vi "PC_DAYWISE.vi"(0 "Refnum in":T1, 1 "BREAKDOWN_STK_HOLD_ID":i32=1, 2 "condition":string="Where BREAKDOWN_DATE between '%s'and '%s' and BREAKDOWN_STK_HOLD_ID ='%d'  ", 5 "Form Date":timestamp, 7 "Array":string[](array[string]), 9 "To Date":timestamp, 11 "error in (no error)":errorcluster, 12 "STATION_ID_CID_TRIGGER":i32) -> (4 "Refnum out":T1, 6 "Count out":string[](array[string]), 15 "error out":errorcluster)   [LabVIEW 2017]
uses:
  <vilib>/addons/database/Connection.llb/Conn ObjectReference.ctl
  <vilib>/addons/database/NI_Database_API.lvlib
panel:
  out "subarray":string[](array[string])
  out "Table":string[][](array[string])
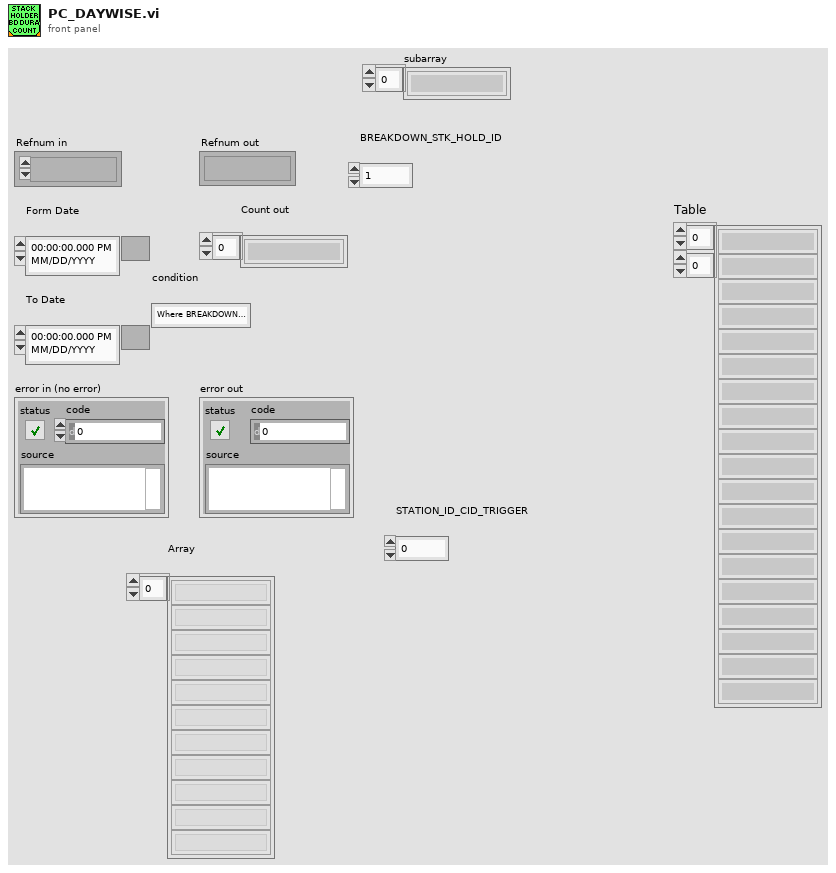
[diagram p1: front panel]
types:
  T1 = typedef "NI_Database_API.lvlib/Conn ObjectReference.ctl" = refnum<k1>
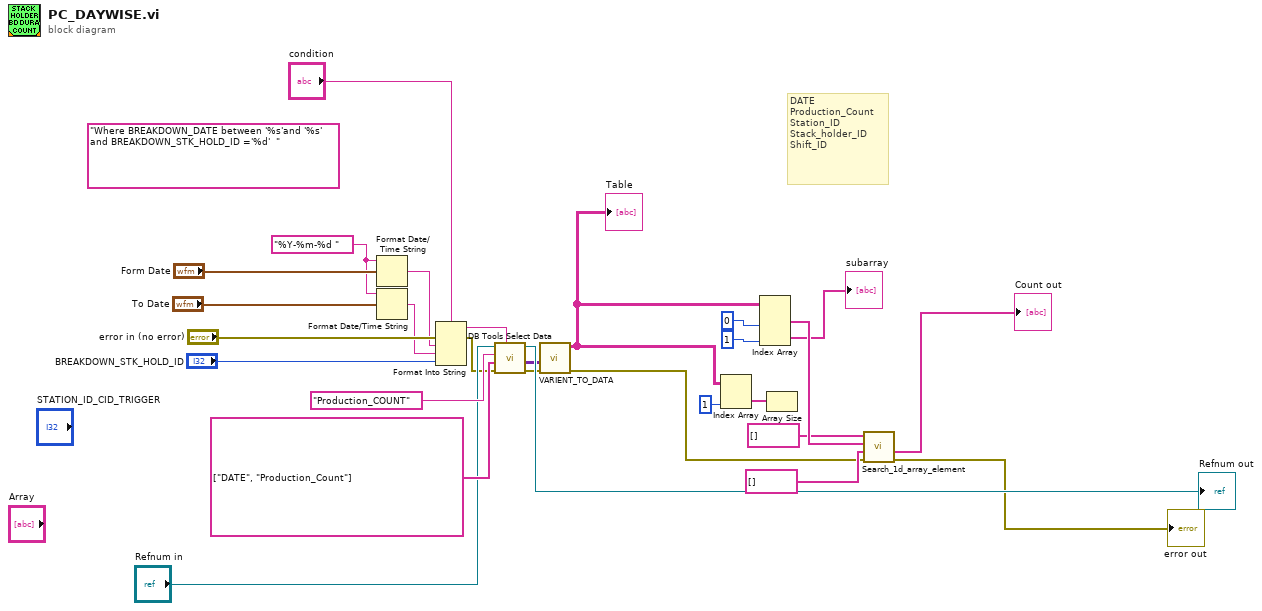
[diagram p0: block diagram]
diagram:
  (unwired) "Where BREAKDOWN_DATE between '%s'and '%s' and BREAKDOWN_STK_HOLD_ID ='%d'  "
  w9 = "%Y-%m-%d " ("time format string (%c)")
  # "DATE\nProduction_Count\nStation_ID\nStack_holder_ID\nShift_ID"
  n1 = Format Date/Time String(time format string (%c)=w9, seconds (now)="Form Date") -> (date/time string=w12:string)  [unwired: 1 in]
  n2 = Format Date/Time String(time format string (%c)=w9, seconds (now)="To Date") -> (date/time string=w13:string)  [unwired: 1 in]
  n3 = Format Into String(format string="condition", error in="error in (no error)", w12, w13, "BREAKDOWN_STK_HOLD_ID") -> (resulting string=w5:string, error out=w6:errorcluster)  [unwired: 1 in]
  n4 = call <vilib>:"DB Tools Select Data.vi"("condition"=w5, "error in (no error)"=w6, "columns"=string[] ["DATE", "Production_Count"], "table"="Production_COUNT", "connection reference"="Refnum in") -> ("error out"=w7:errorcluster, "data"=w8:variant[][], "connection reference out"=→"Refnum out":T1)  [unwired: 1 in]
  n5 = call "VARIENT_TO_DATA.vi"("data"=w8, "error in (no error)"=w7) -> ("Table"=w26:string[][], "error out"=w27:errorcluster)  [unwired: 7 in]
  "Table" <- w26
  n6 = Index Array(array=w26, index (col)=1 ("disabled index (col)")) -> (element=w23:string[])  [unwired: 1 in]
  n7 = Index Array(array=w26, index (col) #1=0 ("disabled index (col)"), index (col) #2=1 ("disabled index (col)")) -> (element #1=w25:string[], element #2=→"subarray":string[])  [unwired: 2 in]
  n8 = Array Size(array=w23) -> ()  [unwired: 1 out]
  n9 = call "Search_1d_array_element.vi"("error in (no error)"=w27, "Count in"=string[] [] ("Count"), "BD Date"=w25, "Elements Found in"=string[] [] ("Elements Found")) -> ("error out"=→"error out":errorcluster, "Count out"=→"Count out":string[])  [unwired: 3 in, 1 out]
